vi "Fdx Set Call Library Path.vi"() -> (3 "DllPath":path=path "aim_fdx.19.dll")   [LabVIEW 2020, in "AIM664LV.lvlib"]
doc: "Defines the location of the dynamic library in the specific OS."
uses:
  AIM664LV.lvlib
  FdxGlobalDllPath.vi
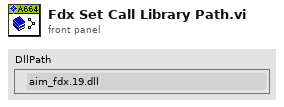
[diagram p1: front panel]
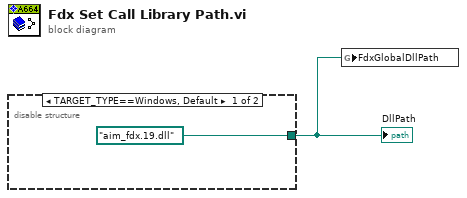
[diagram p0: block diagram]
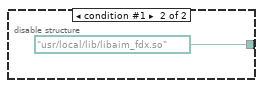
[diagram p2: hidden frame]
diagram:
  n1 = disable-structure "Conditional Disable Structure" shown="TARGET_TYPE==Windows, Default" {
    disable-tunnel: [path "aim_fdx.19.dll" ("GlobalDLLPath") path "/usr/local/lib/libaim_fdx.so" ("DLL Path (if required)")] -> w1
    frame condition #0 (active) {
    }
    frame condition #1 {
    }
  }
  "DllPath" <- w1
  n2 = global write "FdxGlobalDllPath.vi" "FdxGlobalDllPath"(w1) -> ()
